vi "Periodic Tasks.vi"(8 "error in":errorcluster) -> ()   [LabVIEW 2017]
doc: "This VI runs in parallel to other tasks. It can contain as many user-defined periodic loops as you need. These can carry out PID or other sorts of timed response."
uses:
  <vilib>/Rock Robotics/WPI/ThirdParty/Sensors/navX/_TypeDefs/FRIC_navX_DeviceNumbersTypeDef.ctl
  Robot Global Data.vi
  <vilib>/Rock Robotics/Network Tables/NT Write Number.vi
  <vilib>/Rock Robotics/WPI/ThirdParty/Phoenix-LabVIEW/Motor Controller/Get/CTRE_Phoenix_MotorController_GetQuadratureData.vi
  <vilib>/Rock Robotics/WPI/Solenoid/WPI_SolenoidValue.ctl
  <vilib>/Rock Robotics/WPI/Solenoid/WPI_SolenoidSetEnum.vi
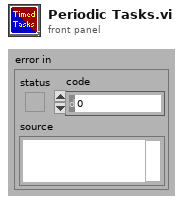
[diagram p1: front panel]
types:
  T1 = typedef "WPI_SolenoidValue.ctl" = enum16{"Off", "On", "Forward", "Reverse"}
  T2 = typedef "WPI_SolenoidDevRef.ctl" = cluster{"DevStatus":errorcluster, "Pneumatics Control Module":u8, "Forward Solenoid Channel":T3, "Reverse Solenoid Channel":T3}
  T3 = typedef "WPI_SolenoidChannel.ctl" = enum8{"Solenoid 0", "Solenoid 1", "Solenoid 2", "Solenoid 3", "Solenoid 4", "Solenoid 5", "Solenoid 6", "Solenoid 7", "Invalid"}
  T4 = typedef "WPI_MotorControlDeviceRef.ctl" = cluster{"DeviceStatus":errorcluster, "Type":T5, "PWM":cluster{"PWM Channel":T6, "DeadBand":T7}, "CAN":cluster{"Device Number":u8, "SetOutput VI Ref":variant, "GetOutput VI Ref":variant, "Enable VI Ref":variant, "Disable VI Ref":variant, "Data":variant}, "Invert":bool, "DIO PWM":cluster{"PWM \"Enable\" Channel":T6, "DIOChannel":T8, "PWM Rate":dbl}}
  T5 = typedef "WPI_MotorControlType.ctl" = enum16{"PWM", "CAN", "DIO PWM"}
  T6 = typedef "FPGA_DIOPWMChannel.ctl" = enum8{"PWM 0", "PWM 1", "PWM 2", "PWM 3", "PWM 4", "PWM 5", "PWM 6", "PWM 7", "PWM 8", "PWM 9", "PWM MXP 0", "PWM MXP 1", "PWM MXP 2", "PWM MXP 3", "PWM MXP 4", "PWM MXP 5", "PWM MXP 6", "PWM MXP 7", "PWM MXP 8", "PWM MXP 9", "Invalid"}
  T7 = typedef "WPI_PWMDeadband.ctl" = cluster{"Name":string, "maxPositivePwm":i32, "minPositivePwm":i32, "centerPwm":i32, "maxNegativePwm":i32, "minNegativePwm":i32, "angularRange":u16}
  T8 = typedef "FPGA_DIOChannel.ctl" = enum8{"DIO 0", "DIO 1", "DIO 2", "DIO 3", "DIO 4", "DIO 5", "DIO 6", "DIO 7", "DIO 8", "DIO 9", "DIO MXP 0", "DIO MXP 1", "DIO MXP 2", "DIO MXP 3", "DIO MXP 4", "DIO MXP 5", "DIO MXP 6", "DIO MXP 7", "DIO MXP 8", "DIO MXP 9", "DIO MXP 10", "DIO MXP 11", "DIO MXP 12", "DIO MXP 13", "DIO MXP 14", "DIO MXP 15", "SPI Port CS1", "SPI Port CS2", "SPI Port CS3", "SPI Port MISO", "SPI Port MOSI", "Invalid"}
  T9 = typedef "FRIC_navX_DeviceNumbersTypeDef.ctl" = enum16{"Dev0", "Dev1", "Dev2", "Dev3"}
  T10 = cluster{"Yaw":dbl, "Roll":dbl, "Pitch":dbl, "Heading":dbl, "Fused Heading":dbl}
  T11 = typedef "WPI_RobotDriveDevRef.ctl" = cluster{"DevStatus":errorcluster, "Motors[]":T4[], "Square Inputs":bool, "Max Output":dbl}
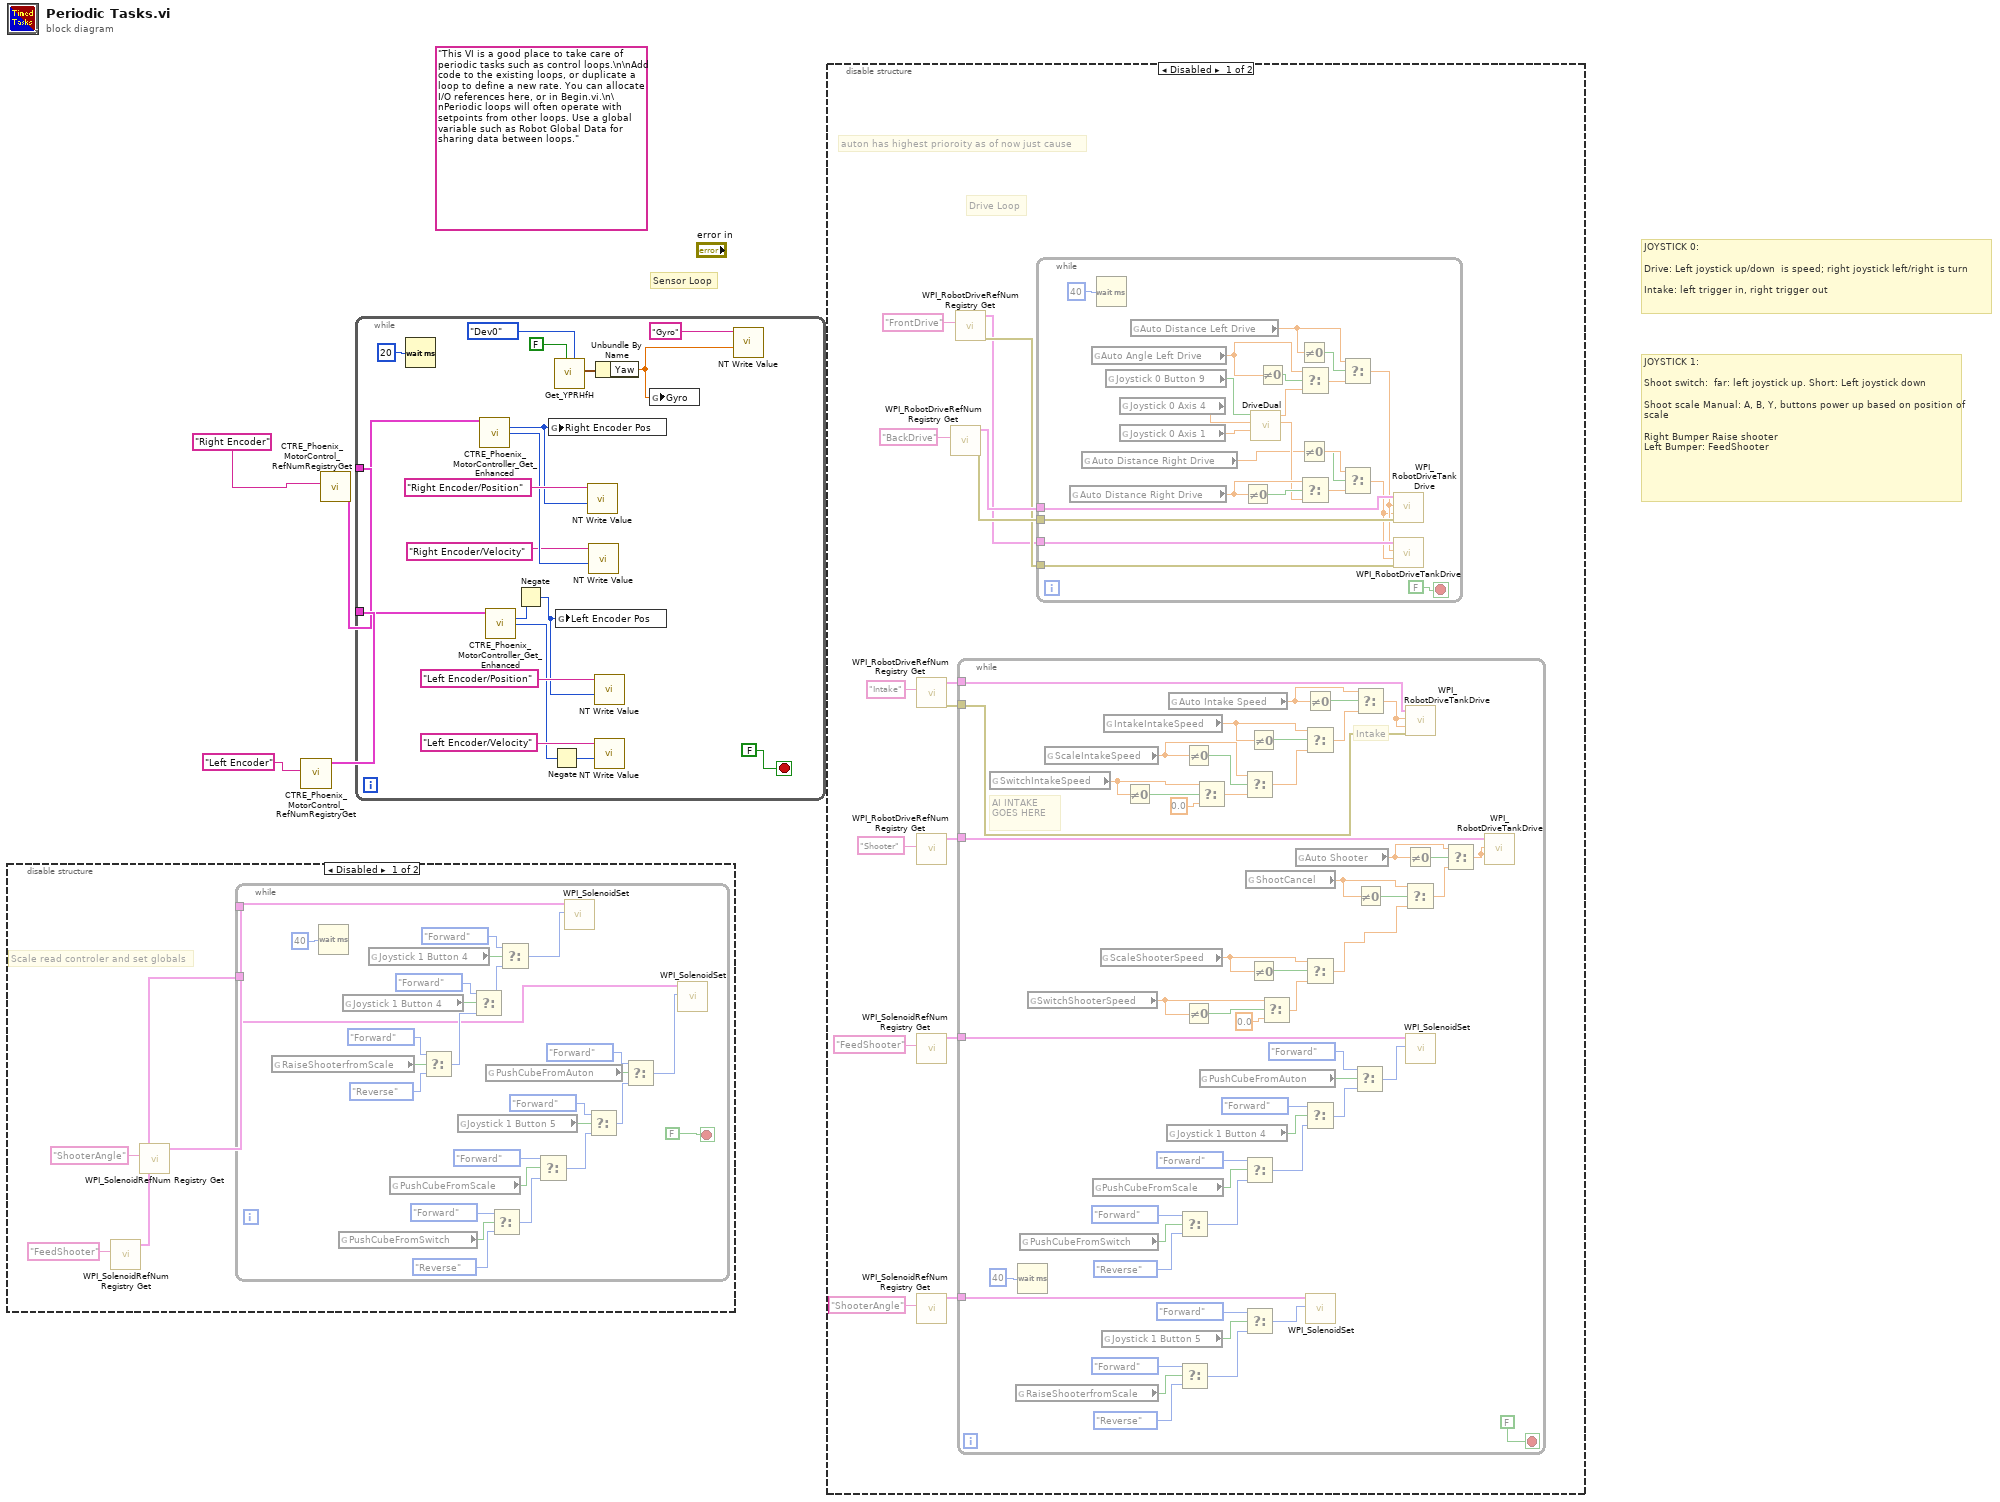
[diagram p0: block diagram]
diagram:
  (unwired) "This VI is a good place to take care of periodic tasks such as control loops.\n\nAdd code to the existing loops, or duplicate a loop to define a new rate. You can allocate I/O references here, or in Begin.vi.\n\nPeriodic loops will often operate with setpoints from other loops. Use a global variable such as Robot Global Data for sharing data between loops."
  # "Sensor Loop"
  # "JOYSTICK 1:\n\nShoot switch:  far: left joystick up. Short: Left joystick down\n\nShoot scale Manual: A, B, Y, buttons power up based on position of scale\n\nRight Bumper Raise shooter\nLeft Bumper: FeedShooter"
  # "JOYSTICK 0:\n\nDrive: Left joystick up/down  is speed; right joystick left/right is turn\n\nIntake: left trigger in, right trigger out"
  n1 = disable-structure shown="Disabled" {
    frame Disabled {
      # "Scale read controler and set globals"
      n2 = call <vilib>:"WPI_SolenoidRefNum Registry Get.vi"("refnum name"="FeedShooter") -> ("SolenoidDevRef"=w6:T2)  [unwired: 9 in, 1 out]
      n3 = call <vilib>:"WPI_SolenoidRefNum Registry Get.vi"("refnum name"="ShooterAngle") -> ("SolenoidDevRef"=w7:T2)  [unwired: 9 in, 1 out]
      n4 = while {
        tunnel: w7 -> [w18]
        tunnel: w6 -> [w17]
        stop <- FALSE stop-if-true
        n5 = global read "Robot Global Data.vi" "RaiseShooterfromScale"() -> (w28:bool)
        n6 = Wait (ms)(milliseconds to wait=u32 40) -> ()  [unwired: 1 out]
        n7 = global read "Robot Global Data.vi" "PushCubeFromSwitch"() -> (w22:bool)
        n8 = global read "Robot Global Data.vi" "Joystick 1 Button 4"() -> (w30:bool)
        n9 = global read "Robot Global Data.vi" "Joystick 1 Button 4"() -> (w12:bool)
        n10 = global read "Robot Global Data.vi" "PushCubeFromScale"() -> (w24:bool)
        n11 = Select(t=WPI_SolenoidValue."Forward" ("Value"), s=w28, f=WPI_SolenoidValue."Reverse" ("Value")) -> (s? t:f=w29:T1)
        n12 = global read "Robot Global Data.vi" "Joystick 1 Button 5"() -> (w33:bool)
        n13 = Select(t=WPI_SolenoidValue."Forward" ("Value"), s=w30, f=w29) -> (s? t:f=w10:T1)
        n14 = global read "Robot Global Data.vi" "PushCubeFromAuton"() -> (w15:bool)
        n15 = Select(t=WPI_SolenoidValue."Forward" ("Value"), s=w22, f=WPI_SolenoidValue."Reverse" ("Value")) -> (s? t:f=w21:T1)
        n16 = Select(t=WPI_SolenoidValue."Forward" ("Value"), s=w12, f=w10) -> (s? t:f=w9:T1)
        n17 = Select(t=WPI_SolenoidValue."Forward" ("Value"), s=w24, f=w21) -> (s? t:f=w26:T1)
        n18 = call-poly <vilib>:"WPI_SolenoidSet.vi"("Value"=w9, "SolenoidDevRef"=w18) -> ()  [unwired: 8 in, 2 out]
        n19 = Select(t=WPI_SolenoidValue."Forward" ("Value"), s=w33, f=w26) -> (s? t:f=w14:T1)
        n20 = Select(t=WPI_SolenoidValue."Forward" ("Value"), s=w15, f=w14) -> (s? t:f=w13:T1)
        n21 = call-poly <vilib>:"WPI_SolenoidSet.vi"("Value"=w13, "SolenoidDevRef"=w17) -> ()  [unwired: 8 in, 2 out]
      }
    }
    frame Enabled {
    }
  }
  n22 = call <vilib>:"CTRE_Phoenix_MotorControl_RefNumRegistryGet.vi"("refnum name"="Left Encoder") -> ("PhoenixMotorControlDevRef"=w4:T4)  [unwired: 9 in, 1 out]
  n23 = call <vilib>:"CTRE_Phoenix_MotorControl_RefNumRegistryGet.vi"("refnum name"="Right Encoder") -> ("PhoenixMotorControlDevRef"=w1:T4)  [unwired: 9 in, 1 out]
  n24 = while {
    tunnel: w4 -> [w52]
    tunnel: w1 -> [w45]
    stop <- FALSE stop-if-true
    n25 = Wait (ms)(milliseconds to wait=u32 20) -> ()  [unwired: 1 out]
    n26 = call-poly <vilib>:"CTRE_Phoenix_MotorController_Get_Enhanced.vi"("PhoenixMotorControlDevRef"=w45) -> ("Quadrature Position"=w40:i32, "Quadrature Velocity"=w43:i32)  [unwired: 11 in, 2 out]
    n27 = call-poly <vilib>:"CTRE_Phoenix_MotorController_Get_Enhanced.vi"("PhoenixMotorControlDevRef"=w52) -> ("Quadrature Position"=w39:i32, "Quadrature Velocity"=w37:i32)  [unwired: 11 in, 2 out]
    n28 = Negate(x=w39) -> (-x=w38:i32)
    n29 = global write "Robot Global Data.vi" "Right Encoder Pos"(w40) -> ()
    n30 = Negate(x=w37) -> (-x=w36:i32)
    n31 = call <vilib>:"Get_YPRHfH.vi"("Device Number"=FRIC_navX_DeviceNumbersTypeDef."Dev0", "Update"=FALSE) -> ("YRPHfH"=w48:T10)  [unwired: 9 in]
    n32 = global write "Robot Global Data.vi" "Left Encoder Pos"(w38) -> ()
    n33 = call-poly <vilib>:"NT Write Value.vi"("Numeric"=w40, "Name"="Right Encoder/Position") -> ()  [unwired: 9 in, 1 out]
    n34 = call-poly <vilib>:"NT Write Value.vi"("Numeric"=w43, "Name"="Right Encoder/Velocity") -> ()  [unwired: 9 in, 1 out]
    n35 = call-poly <vilib>:"NT Write Value.vi"("Numeric"=w38, "Name"="Left Encoder/Position") -> ()  [unwired: 9 in, 1 out]
    n36 = call-poly <vilib>:"NT Write Value.vi"("Numeric"=w36, "Name"="Left Encoder/Velocity") -> ()  [unwired: 9 in, 1 out]
    n37 = Unbundle By Name(w48) -> ("Yaw"=w41:dbl)
    n38 = global write "Robot Global Data.vi" "Gyro"(w41) -> ()
    n39 = call-poly <vilib>:"NT Write Value.vi"("Numeric"=w41, "Name"="Gyro") -> ()  [unwired: 9 in, 1 out]
  }
  n40 = disable-structure shown="Disabled" {
    frame Disabled {
      # "auton has highest prioroity as of now just cause"
      # "Drive Loop"
      n41 = call <vilib>:"WPI_RobotDriveRefNum Registry Get.vi"("refnum name"="Intake") -> ("error out"=w62:errorcluster, "RobotDriveDevRef"=w61:T11)  [unwired: 9 in]
      n42 = call <vilib>:"WPI_RobotDriveRefNum Registry Get.vi"("refnum name"="Shooter") -> ("RobotDriveDevRef"=w59:T11)  [unwired: 9 in, 1 out]
      n43 = call <vilib>:"WPI_SolenoidRefNum Registry Get.vi"("refnum name"="FeedShooter") -> ("SolenoidDevRef"=w56:T2)  [unwired: 9 in, 1 out]
      n44 = call <vilib>:"WPI_SolenoidRefNum Registry Get.vi"("refnum name"="ShooterAngle") -> ("SolenoidDevRef"=w55:T2)  [unwired: 9 in, 1 out]
      n45 = call <vilib>:"WPI_RobotDriveRefNum Registry Get.vi"("refnum name"="BackDrive") -> ("error out"=w68:errorcluster, "RobotDriveDevRef"=w67:T11)  [unwired: 9 in]
      n46 = call <vilib>:"WPI_RobotDriveRefNum Registry Get.vi"("refnum name"="FrontDrive") -> ("error out"=w65:errorcluster, "RobotDriveDevRef"=w64:T11)  [unwired: 9 in]
      n47 = while {
        tunnel: w62 -> [w106]
        tunnel: w61 -> [w105]
        tunnel: w59 -> [w104]
        tunnel: w56 -> [w73]
        tunnel: w55 -> [w72]
        stop <- FALSE stop-if-true
        # "AI INTAKE GOES HERE"
        # "Intake"
        n48 = global read "Robot Global Data.vi" "SwitchIntakeSpeed"() -> (w120:dbl)
        n49 = global read "Robot Global Data.vi" "RaiseShooterfromScale"() -> (w87:bool)
        n50 = Wait (ms)(milliseconds to wait=u32 40) -> ()  [unwired: 1 out]
        n51 = global read "Robot Global Data.vi" "PushCubeFromSwitch"() -> (w81:bool)
        n52 = global read "Robot Global Data.vi" "SwitchShooterSpeed"() -> (w108:dbl)
        n53 = global read "Robot Global Data.vi" "ScaleIntakeSpeed"() -> (w116:dbl)
        n54 = global read "Robot Global Data.vi" "PushCubeFromScale"() -> (w83:bool)
        n55 = global read "Robot Global Data.vi" "ScaleShooterSpeed"() -> (w112:dbl)
        n56 = global read "Robot Global Data.vi" "Joystick 1 Button 5"() -> (w89:bool)
        n57 = global read "Robot Global Data.vi" "IntakeIntakeSpeed"() -> (w114:dbl)
        n58 = Not Equal To 0?(x=w120) -> (x != 0?=w121:bool)
        n59 = global read "Robot Global Data.vi" "Joystick 1 Button 4"() -> (w92:bool)
        n60 = global read "Robot Global Data.vi" "Auto Intake Speed"() -> (w103:dbl)
        n61 = Select(t=WPI_SolenoidValue."Forward" ("Value"), s=w81, f=WPI_SolenoidValue."Reverse" ("Value")) -> (s? t:f=w80:T1)
        n62 = Select(t=WPI_SolenoidValue."Forward" ("Value"), s=w87, f=WPI_SolenoidValue."Reverse" ("Value")) -> (s? t:f=w88:T1)
        n63 = Not Equal To 0?(x=w116) -> (x != 0?=w117:bool)
        n64 = Not Equal To 0?(x=w108) -> (x != 0?=w107:bool)
        n65 = Select(t=w120, s=w121, f=0.0) -> (s? t:f=w118:dbl)
        n66 = global read "Robot Global Data.vi" "PushCubeFromAuton"() -> (w76:bool)
        n67 = Select(t=w116, s=w117, f=w118) -> (s? t:f=w113:dbl)
        n68 = Select(t=WPI_SolenoidValue."Forward" ("Value"), s=w83, f=w80) -> (s? t:f=w85:T1)
        n69 = Select(t=WPI_SolenoidValue."Forward" ("Value"), s=w89, f=w88) -> (s? t:f=w71:T1)
        n70 = global read "Robot Global Data.vi" "ShootCancel"() -> (w99:dbl)
        n71 = Not Equal To 0?(x=w114) -> (x != 0?=w115:bool)
        n72 = Not Equal To 0?(x=w112) -> (x != 0?=w111:bool)
        n73 = Select(t=w108, s=w107, f=0.0) -> (s? t:f=w110:dbl)
        n74 = global read "Robot Global Data.vi" "Auto Shooter"() -> (w96:dbl)
        n75 = Not Equal To 0?(x=w103) -> (x != 0?=w102:bool)
        n76 = Select(t=w114, s=w115, f=w113) -> (s? t:f=w101:dbl)
        n77 = Select(t=w112, s=w111, f=w110) -> (s? t:f=w70:dbl)
        n78 = Select(t=WPI_SolenoidValue."Forward" ("Value"), s=w92, f=w85) -> (s? t:f=w75:T1)
        n79 = call-poly <vilib>:"WPI_SolenoidSet.vi"("Value"=w71, "SolenoidDevRef"=w72) -> ()  [unwired: 8 in, 2 out]
        n80 = Select(t=WPI_SolenoidValue."Forward" ("Value"), s=w76, f=w75) -> (s? t:f=w74:T1)
        n81 = Select(t=w103, s=w102, f=w101) -> (s? t:f=w100:dbl)
        n82 = Not Equal To 0?(x=w99) -> (x != 0?=w98:bool)
        n83 = Not Equal To 0?(x=w96) -> (x != 0?=w97:bool)
        n84 = Select(t=w99, s=w98, f=w70) -> (s? t:f=w94:dbl)
        n85 = call <vilib>:"WPI_RobotDriveTankDrive.vi"("error in (no error)"=w106, "Right axis value"=w100, "Left axis value"=w100, "RobotDriveDevRef"=w105) -> ()  [unwired: 5 in, 3 out]
        n86 = call-poly <vilib>:"WPI_SolenoidSet.vi"("Value"=w74, "SolenoidDevRef"=w73) -> ()  [unwired: 8 in, 2 out]
        n87 = Select(t=w96, s=w97, f=w94) -> (s? t:f=w95:dbl)
        n88 = call <vilib>:"WPI_RobotDriveTankDrive.vi"("Right axis value"=w95, "Left axis value"=w95, "RobotDriveDevRef"=w104) -> ()  [unwired: 6 in, 3 out]
      }
      n89 = while {
        tunnel: w68 -> [w135]
        tunnel: w67 -> [w134]
        tunnel: w65 -> [w133]
        tunnel: w64 -> [w132]
        stop <- FALSE stop-if-true
        n90 = global read "Robot Global Data.vi" "Auto Distance Right Drive"() -> (w139:dbl)
        n91 = global read "Robot Global Data.vi" "Auto Distance Right Drive"() -> (w126:dbl)
        n92 = global read "Robot Global Data.vi" "Auto Angle Left Drive"() -> (w140:dbl)
        n93 = Wait (ms)(milliseconds to wait=u32 40) -> ()  [unwired: 1 out]
        n94 = global read "Robot Global Data.vi" "Joystick 0 Button 9"() -> (w131:bool)
        n95 = global read "Robot Global Data.vi" "Joystick 0 Axis 4"() -> (w142:dbl)
        n96 = global read "Robot Global Data.vi" "Joystick 0 Axis 1"() -> (w143:dbl)
        n97 = global read "Robot Global Data.vi" "Auto Distance Left Drive"() -> (w130:dbl)
        n98 = Not Equal To 0?(x=w139) -> (x != 0?=w138:bool)
        n99 = call "DriveDual.vi"("YAxis"=w143, "XAxis"=w142, "Turbo?"=w131) -> ("Right"=w137:dbl, "Left"=w136:dbl)  [unwired: 7 in]
        n100 = Not Equal To 0?(x=w140) -> (x != 0?=w141:bool)
        n101 = Not Equal To 0?(x=w130) -> (x != 0?=w129:bool)
        n102 = Not Equal To 0?(x=w126) -> (x != 0?=w123:bool)
        n103 = Select(t=w140, s=w141, f=w136) -> (s? t:f=w128:dbl)
        n104 = Select(t=w139, s=w138, f=w137) -> (s? t:f=w124:dbl)
        n105 = Select(t=w130, s=w129, f=w128) -> (s? t:f=w127:dbl)
        n106 = Select(t=w126, s=w123, f=w124) -> (s? t:f=w125:dbl)
        n107 = call <vilib>:"WPI_RobotDriveTankDrive.vi"("error in (no error)"=w135, "Right axis value"=w125, "Left axis value"=w127, "RobotDriveDevRef"=w134) -> ()  [unwired: 5 in, 3 out]
        n108 = call <vilib>:"WPI_RobotDriveTankDrive.vi"("error in (no error)"=w133, "Right axis value"=w125, "Left axis value"=w127, "RobotDriveDevRef"=w132) -> ()  [unwired: 5 in, 3 out]
      }
    }
    frame Enabled {
    }
  }
